vi "DB Tools Create Parameterized Query.vi"(4 "stored procedure? (F)":bool, 5 "auto-detect parameters? (F)":bool, 6 "error in (no error)":errorcluster, 7 "parameters":T3[](array[typedef]), 8 "SQL query":string, 9 "connection reference":T2) -> (0 "error out":errorcluster, 1 "parameters out":T3[](array[typedef]), 3 "command reference":T6)   [LabVIEW 2012, in "NI_Database_API_64.lvlib"]
doc: "Creates a parameterized <B>SQL query</B> and returns a <B>command reference</B> that you must free eventually. Unless you are detecting the parameters automatically, the number of elements in the <B>parameters</B> array must match the number of parameters you specify in <B>SQL query</B>. For stored procedures, set <B>stored procedure</B> to TRUE and <B>SQL query</B> to the name of the procedure you want to execute."
uses:
  NI_Database_API_64.lvlib
  Connection.llb/Conn ObjectReference.ctl
  Cmd ObjectReference.ctl
  Cmd DataMembers.ctl
  Auxilliary.llb/DB Tools Parameter Info.ctl
  Auxilliary.llb/DB Tools DataTypes.ctl
  Auxilliary.llb/DB Tools Parameter Dir.ctl
  Connection.llb/Conn Get Properties.vi
panel:
  in  "default":T1
  in  "default data":T1
  in  "ADODB._Command":refnum<k7>
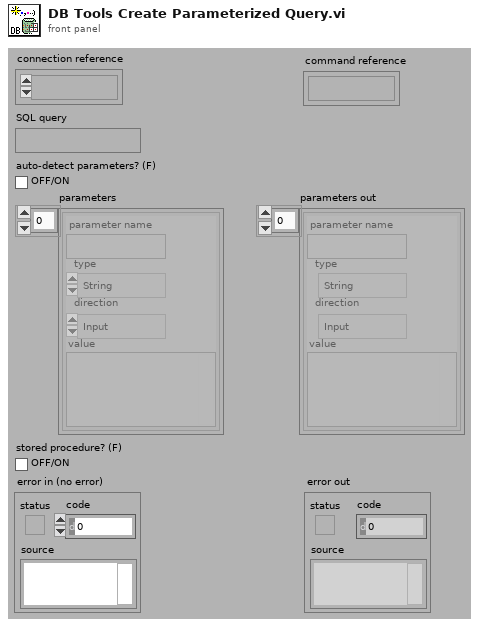
[diagram p1: front panel]
types:
  T1 = typedef "NI_Database_API_64.lvlib/Cmd DataMembers.ctl" = cluster{"ADODB._Command":refnum<k7>, "Connection":T2}
  T2 = typedef "NI_Database_API_64.lvlib/Conn ObjectReference.ctl" = refnum<k1>
  T3 = typedef "NI_Database_API_64.lvlib/DB Tools Parameter Info.ctl" = cluster{"parameter name":string, "type":T4, "direction":T5, "value":variant}
  T4 = typedef "NI_Database_API_64.lvlib/DB Tools DataTypes.ctl" = enum16{"String", "Long (I32)", "Single (SGL)", "Double (DBL)", "Date/Time", "Binary"}
  T5 = typedef "NI_Database_API_64.lvlib/DB Tools Parameter Dir.ctl" = enum32{"Input", "Output", "Input/Output", "Return Value"}
  T6 = typedef "NI_Database_API_64.lvlib/Cmd ObjectReference.ctl" = refnum<k1>
  T7 = typedef "NI_Database_API_64.lvlib/Conn Properties.ctl" = cluster{"command timeout (s)":i32, "connection string":string, "default database":string, "provider":string}
  T8 = typedef "NI_Database_API_64.lvlib/Conn DataMembers.ctl" = cluster{"ADODB._Connection":refnum<k7>, "recordset objects":i32, "command objects":i32}
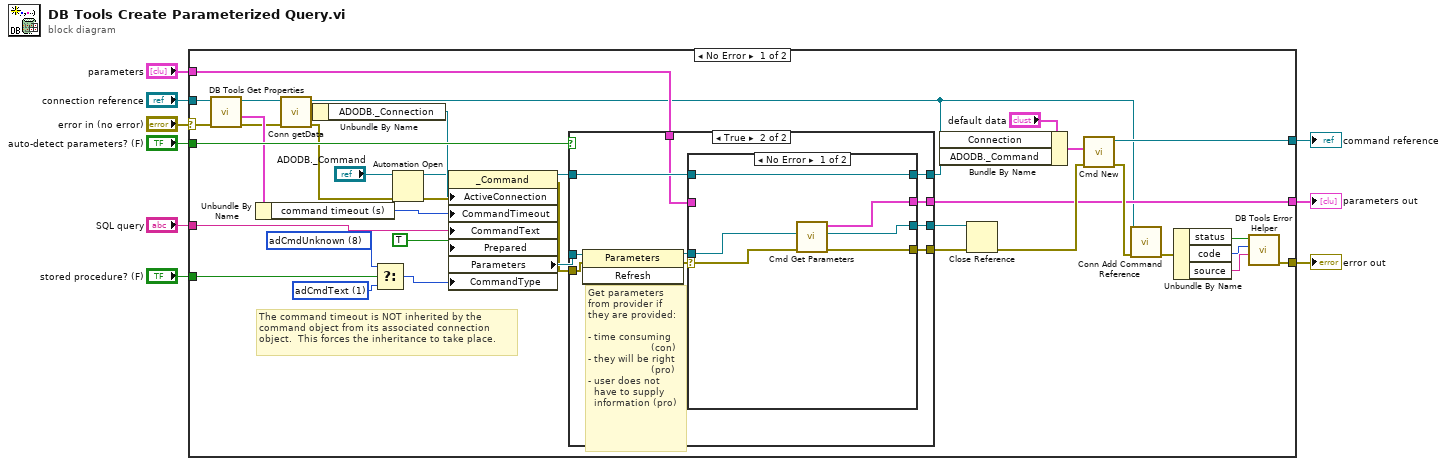
[diagram p0: block diagram]
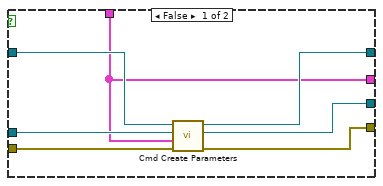
[diagram p2: hidden frame]
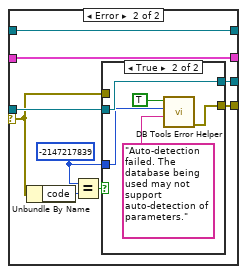
[diagram p3: hidden frame]
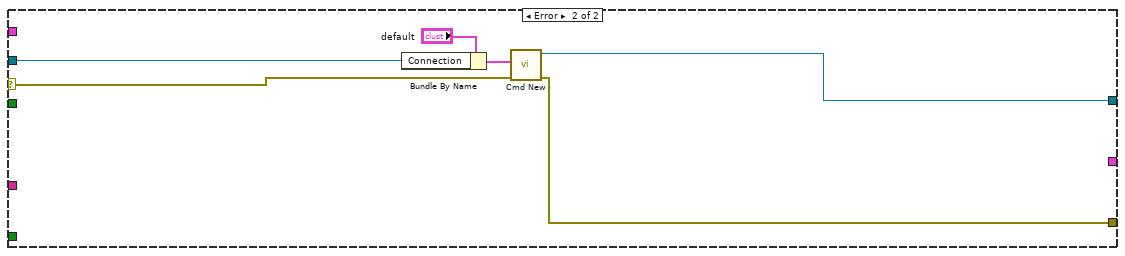
[diagram p5: hidden frame]
diagram:
  n1 = case shown="No Error" "error in (no error)" {
    selector: "error in (no error)" -> [w10 w90]
    tunnel: "stored procedure? (F)" -> [w47 _]
    tunnel: [w42 w87] -> w8
    tunnel: "auto-detect parameters? (F)" -> [w41 _]
    tunnel: "connection reference" -> [w34 w88]
    tunnel: "SQL query" -> [w33 _]
    tunnel: "parameters" -> [w27 _]
    tunnel: [w26 _] -> w3
    tunnel: [w16 w89] -> w2
    frame No Error {
      w45 = 1 items=["adCmdUnspecified"=-1, "adCmdUnknown"=8, "adCmdText"=1, "adCmdTable"=2, "adCmdStoredProc"=4, "adCmdFile"=256, "adCmdTableDirect"=512] ("CommandType")
      w46 = 8 items=["adCmdUnspecified"=-1, "adCmdUnknown"=8, "adCmdText"=1, "adCmdTable"=2, "adCmdStoredProc"=4, "adCmdFile"=256, "adCmdTableDirect"=512] ("CommandType")
      # "The command timeout is NOT inherited by the \ncommand object from its associated connection \nobject.  This forces the inheritance to take place."
      n2 = call-poly "DB Tools Get Properties.vi"("error in (no error)"=w10, "connection reference"=w34) -> ("error out"=w22:errorcluster, "connection properties"=w28:T7, "connection reference out"=w23:T2)  [unwired: 3 out]
      n3 = Unbundle By Name(w28) -> ("command timeout (s)"=w31:i32)
      n4 = call "Conn getData.vi"("error in (no error)"=w22, "connection reference"=w23) -> ("error out"=w12:errorcluster, "data"=w25:T8, "connection reference out"=w24:T2)  [unwired: 3 out]
      n5 = Unbundle By Name(w25) -> ("ADODB._Connection"=w21:refnum<k7>)
      n6 = Select(t=w46, s=w47, f=w45) -> (s? t:f=w30:i32)
      n7 = Automation Open(error in (no error)=w12, Automation Refnum="ADODB._Command") -> (Automation Refnum=w13:refnum<k7>, error out=w15:errorcluster)  [unwired: 2 out]
      n8 = property class="_Command"(reference=w13, error in=w15, "ActiveConnection"=w21, "CommandTimeout"=w31, "CommandText"=w33, "Prepared"=TRUE, "CommandType"=w30) -> (reference out=w44:refnum<k7>, error out=w11:errorcluster, "Parameters"=w32:refnum<k7>)
      n9 = case shown="True" w41 {
        tunnel: w32 -> [w52 w64]
        tunnel: w11 -> [w53 w63]
        tunnel: w44 -> [w54 w61]
        tunnel: [w51 w57] -> w36
        tunnel: w27 -> [w49 w58]
        tunnel: [w50 w59] -> w38
        tunnel: [w49 w56] -> w26
        tunnel: [w48 w55] -> w37
        frame False {
          n10 = call "Cmd Create Parameters.vi"("error in (no error)"=w53, "parameters"=w49, "ADODB.Parameters"=w52, "ADODB._Command"=w54) -> ("error out"=w51:errorcluster, "ADODB.Parameters out"=w48:refnum<k7>, "ADODB._Command out"=w50:refnum<k7>)  [unwired: 1 out]
        }
        frame True {
          # "Get parameters \nfrom provider if\nthey are provided:\n\n- time consuming \n                     (con)\n- they will be right \n                     (pro)\n- user does not \n  have to supply\n  information (pro)"
          n11 = invoke class="Parameters" method="Refresh"(reference=w64, error in=w63) -> (reference out=w60:refnum<k7>, error out=w62:errorcluster)  [unwired: 1 in, 1 out]
          n12 = case shown="No Error" w62 {
            selector: w62 -> [w70 w77]
            tunnel: w61 -> [w69 w74]
            tunnel: w60 -> [w66 w78]
            tunnel: [w69 w74] -> w59
            tunnel: w58 -> [_ w75]
            tunnel: [w68 w76] -> w57
            tunnel: [w65 w75] -> w56
            tunnel: [w67 w73] -> w55
            frame No Error {
              n13 = call "Cmd Get Parameters.vi"("error in (no error)"=w70, "ADODB.Parameters"=w66) -> ("error out"=w68:errorcluster, "ADODB.Parameters out"=w67:refnum<k7>, "parameters"=w65:T3[])  [unwired: 1 in, 2 out]
            }
            frame Error {
              w71 = -2147217839
              n14 = Unbundle By Name(w77) -> ("code"=w72:i32)
              n15 = Equal?(x=w71, y=w72) -> (x = y?=w79:bool)
              n16 = case shown="True" w79 {
                tunnel: w78 -> [w80 w86]
                tunnel: w77 -> [w81 _]
                tunnel: [w81 w84] -> w76
                tunnel: [w80 w86] -> w73
                tunnel: w71 -> [_ w83]
                frame False {
                  # "some other error - \ndo nothing and \npass it through"
                }
                frame True {
                  n17 = call "DB Tools Error Helper.vi"("source"="Auto-detection failed. The database being used may not support auto-detection of parameters.", "code"=w83, "status"=TRUE) -> ("error out"=w84:errorcluster)  [unwired: 1 in, 7 out]
                }
              }
            }
          }
        }
      }
      n18 = Bundle By Name(cluster="default data", "Connection"=w24, "ADODB._Command"=w38) -> (w43:T1)
      n19 = Close Reference(reference=w37, error in (no error)=w36) -> (error out=w35:errorcluster)
      n20 = call "Cmd New.vi"("error in (no error)"=w35, "initial data"=w43) -> ("error out"=w39:errorcluster, "command reference"=w42:T6)  [unwired: 4 out]
      n21 = call "Conn Add Command Reference.vi"("error in (no error)"=w39, "connection reference"=w24) -> ("error out"=w17:errorcluster)  [unwired: 9 out]
      n22 = Unbundle By Name(w17) -> ("status"=w19:bool, "code"=w18:i32, "source"=w20:string)
      n23 = call "DB Tools Error Helper.vi"("source"=w20, "code"=w18, "status"=w19) -> ("error out"=w16:errorcluster)  [unwired: 1 in, 7 out]
    }
    frame Error {
      n24 = Bundle By Name(cluster="default", "Connection"=w88) -> (w92:T1)
      n25 = call "Cmd New.vi"("error in (no error)"=w90, "initial data"=w92) -> ("error out"=w89:errorcluster, "command reference"=w87:T6)  [unwired: 4 out]
    }
  }
  "command reference" <- w8
  "error out" <- w2
  "parameters out" <- w3
